vi "Actor Core.vi"(8 "error in":errorcluster, 11 "Sample Photosensor PID Flowsensor PID in":refnum<class "Sample Photosensor PID Flowsensor PID.lvclass">) -> (0 "error out":errorcluster, 3 "Actor out":refnum<class "Actor.lvclass">)   [LabVIEW 2023, in "Sample Photosensor PID Flowsensor PID.lvlib" / "Sample Photosensor PID Flowsensor PID.lvclass"]
doc: "(<B>Filename</B>: Actor Framework.lvlib:Actor.lvclass:Actor Core.vi)\n\nReceives messages to the actor, reacts to them, and initiates any error handling that may shut the actor down.\n\nDescendant classes may override this VI to append parallel tasks for the actor to complete while it handles messages. Overrides use the Call Parent Class Method node."
uses:
  Sample Photosensor PID Flowsensor PID.lvclass
  <vilib>/ActorFramework/Actor/Actor.lvclass
  Sample Photosensor PID Flowsensor PID.lvclass/Sample Photosensor PID Flowsensor PID.ctl
  Series/Series Actor/Series Actor/Series Actor.lvclass/Series Actor.ctl
  <vilib>/ActorFramework/Actor/Actor.lvclass/Actor.ctl
  <vilib>/ActorFramework/Message Enqueuer/Message Enqueuer.lvclass/Message Enqueuer.ctl
  Series/Series Actor/Series Actor Messages/Update Task Point Data Msg/Update Task Point Data Msg.lvclass/Update Task Point Data Msg.ctl
  <vilib>/ActorFramework/Stop Msg/Stop Msg.lvclass/Stop Msg.ctl
  <vilib>/ActorFramework/Message Enqueuer/Init from Existing Queue.vi
  <vilib>/ActorFramework/Message Enqueuer/Enqueue.vi
  <vilib>/ActorFramework/Message Enqueuer/Enqueue Critical.vi
  Series/Series Actor/Series Actor Messages/Update Task Point Data Msg/Update Task Point Data Msg.lvclass
  Series/ISeries Actor/ISeries Actor Messages/Start Tasks Msg/Start Tasks Msg.lvclass
  <vilib>/ActorFramework/Stop Msg/Stop Msg.lvclass
  Series/ISeries Actor/ISeries Actor Messages/Stop Tasks Msg/Stop Tasks Msg.lvclass
  <vilib>/Utility/LVClass/Get LV Class Name.vi
  <resource>/AFDebug/Generate Trace for Message.vi
  <vilib>/ActorFramework/Message Priority Queue/Priority Enqueue.vi
  Series/Series Actor/Series Actor/Series Actor.lvclass
  <vilib>/ActorFramework/Message Enqueuer/Message Enqueuer.lvclass
panel:
  in  "Setpoint Light":dbl(slide) scale=0.0..2.0
  in  "Setpoint Flow":dbl(knob) scale=0.0..2.0
  out "PWM Lamp":dbl(slide) scale=0.0..10.0
  out "PWM Flow":dbl(knob) scale=0.0..1.0
  in  "Kill Series Button":bool
  in  "Stop Button":bool
  in  "Start Button":bool
  out "Photosensor Chart":dbl(graph)
  out "Flowsensor Chart":dbl(graph)
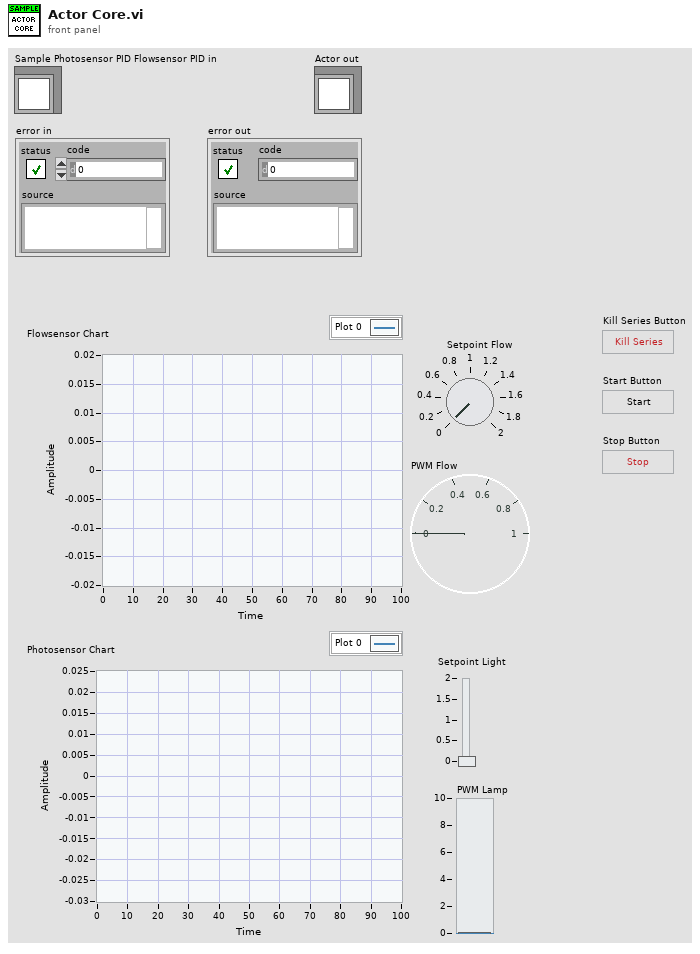
[diagram p1: front panel]
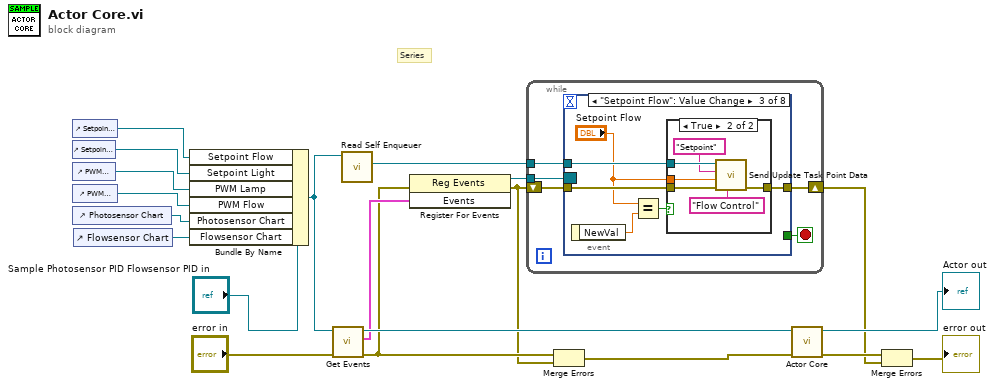
[diagram p0: block diagram]
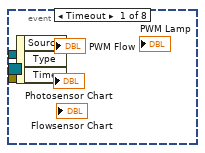
[diagram p2: hidden frame]
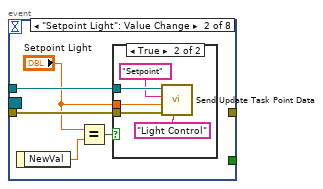
[diagram p3: hidden frame]
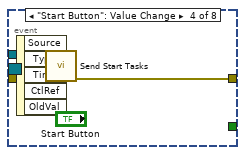
[diagram p6: hidden frame]
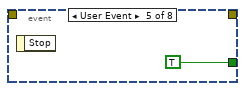
[diagram p7: hidden frame]
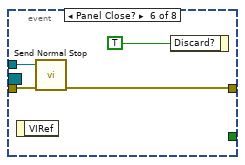
[diagram p8: hidden frame]
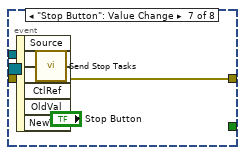
[diagram p9: hidden frame]
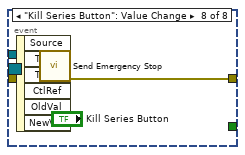
[diagram p10: hidden frame]
diagram:
  # "Series"
  n1 = control-ref of="Setpoint Flow"() -> (w3:refnum<vi>)
  n2 = control-ref of="Setpoint Light"() -> (w2:refnum<vi>)
  n3 = control-ref of="PWM Lamp"() -> (w4:refnum<vi>)
  n4 = control-ref of="PWM Flow"() -> (w5:refnum<vi>)
  n5 = control-ref of="Photosensor Chart"() -> (w7:refnum<vi>)
  n6 = control-ref of="Flowsensor Chart"() -> (w6:refnum<vi>)
  n7 = Bundle By Name(cluster="Sample Photosensor PID Flowsensor PID in", "Setpoint Flow"=w3, "Setpoint Light"=w2, "PWM Lamp"=w4, "PWM Flow"=w5, "Photosensor Chart"=w7, "Flowsensor Chart"=w6) -> (w1:refnum<class "Sample Photosensor PID Flowsensor PID.lvclass">)
  n8 = call "Get Events.vi"("error in (no error)"="error in", "Series Actor in"=w1) -> ("error out"=w12:errorcluster, "Events"=w14:cluster{"Stop":refnum<user-event>}, "Series Actor out"=w15:refnum<class "Sample Photosensor PID Flowsensor PID.lvclass">)  [unwired: 7 in]
  n9 = call <vilib>:"Read Self Enqueuer.vi"("Actor"=w1) -> ("Self Enqueuer"=w17:refnum<class "Message Enqueuer.lvclass">)  [unwired: 10 in]
  n10 = register-events(error in=w12, w14) -> (reference out=w13:refnum<event-registration>, error out=w10:errorcluster)  [unwired: 1 in]
  n11 = while {
    tunnel: w17 -> [w25]
    tunnel: w13 -> [w23]
    shift-right: [w22] -> w8
    shift-left: w10 -> [w24]
    stop <- w21 stop-if-true
    n12 = event shown="[2] \"Setpoint Flow\": Value Change" {
      selector: w23 -> [_ _ _ _ _ _ _ _]
      dyn-events: _ -> [_ _ _ _ _ _ _ _]
      timeout: _ -> [_ _ _ _ _ _ _ _]
      tunnel: w25 -> [_ w30 w37 w51 _ w55 w59 w61]
      tunnel: w24 -> [_ w29 w38 w50 _ w54 w58 w62]
      tunnel: [_ _ w41 w49 _ w53 w57 w60] -> w22
      tunnel: [_ _ _ _ TRUE _ _ _] -> w21
      event Timeout {
        n13 = event-data() -> ()  [unwired: 1 in, 3 out]
      }
      event "Setpoint Light": Value Change {
        n14 = event-data() -> ("NewVal"=w28:dbl)  [unwired: 1 in]
        n15 = Equal?(x="Setpoint Light", y=w28) -> (x = y?=w27:bool)
        n16 = case shown="True" w27 {
          tunnel: w30 -> [_ w35]
          tunnel: w29 -> [_ w34]
          tunnel: "Setpoint Light" -> [_ w31]
          frame False {
          }
          frame True {
            n17 = call "Send Update Task Point Data.vi"("Task Ident"="Light Control", "error in (no error)"=w34, "Data"=w31, "Point Ident"="Setpoint", "Message Enqueuer"=w35) -> ()  [unwired: 5 in, 2 out]
          }
        }
      }
      event "Setpoint Flow": Value Change {
        n18 = event-data() -> ("NewVal"=w39:dbl)  [unwired: 1 in]
        n19 = Equal?(x="Setpoint Flow", y=w39) -> (x = y?=w40:bool)
        n20 = case shown="True" w40 {
          tunnel: w37 -> [_ w48]
          tunnel: w38 -> [w42 w47]
          tunnel: [w42 w44] -> w41
          tunnel: "Setpoint Flow" -> [_ w43]
          frame False {
          }
          frame True {
            n21 = call "Send Update Task Point Data.vi"("Task Ident"="Flow Control", "error in (no error)"=w47, "Data"=w43, "Point Ident"="Setpoint", "Message Enqueuer"=w48) -> ("error out"=w44:errorcluster)  [unwired: 5 in, 1 out]
          }
        }
      }
      event "Start Button": Value Change {
        n22 = event-data() -> ()  [unwired: 1 in, 5 out]
        n23 = call "Send Start Tasks.vi"("error in (no error)"=w50, "Message Enqueuer"=w51) -> ("error out"=w49:errorcluster)  [unwired: 8 in, 1 out]
      }
      event User Event {
        n24 = event-data() -> ()  [unwired: 1 in, 1 out]
      }
      event Panel Close? {
        n25 = event-data() -> ()  [unwired: 1 in, 1 out]
        n26 = call <vilib>:"Send Normal Stop.vi"("error in (no error)"=w54, "Message Enqueuer"=w55) -> ("error out"=w53:errorcluster)  [unwired: 9 in]
        n27 = event-data("Discard?"=TRUE) -> ()  [unwired: 1 in, 1 out]
      }
      event "Stop Button": Value Change {
        n28 = event-data() -> ()  [unwired: 1 in, 6 out]
        n29 = call "Send Stop Tasks.vi"("error in (no error)"=w58, "Message Enqueuer"=w59) -> ("error out"=w57:errorcluster)  [unwired: 8 in, 1 out]
      }
      event "Kill Series Button": Value Change {
        n30 = event-data() -> ()  [unwired: 1 in, 6 out]
        n31 = call <vilib>:"Send Emergency Stop.vi"("error in (no error)"=w62, "Message Enqueuer"=w61) -> ("error out"=w60:errorcluster)  [unwired: 9 in]
      }
    }
  }
  n32 = Merge Errors(w12, w10) -> (w11:errorcluster)
  n33 = call-parent "Actor Core.vi"("error in"=w11, "Series Actor in"=w15) -> ("error out"=w20:errorcluster, "Actor out"=→"Actor out":refnum<class "Actor.lvclass">)  [unwired: 8 in]
  n34 = Merge Errors(w20, w8) -> (→"error out":errorcluster)
